vi "Target3.vi"() -> ()   [LabVIEW 2025]
uses:
  <vilib>/Platform/TimedLoop/XDataNode/timing_clust.ctl
  <vilib>/Platform/TimedLoop/XDataNode/nitl_modes.ctl
  <vilib>/Platform/TimedLoop/XDataNode/wakeup.ctl
  <vilib>/rvi/Emulation/niFpgaSctlEmulationGetInTimedLoop.vi
  <vilib>/rvi/Emulation/niFpgaEmulationReportErrorSimple.vi
  <vilib>/rvi/Emulation/niFpgaGetClockAttributes.vi
  <vilib>/rvi/Emulation/niFpgaCriticalErrorInLSC.vi
  <vilib>/rvi/linearAlgebra/MatrixMultiply/simVIs/SubVI/nifxpla_MatrixMultiply_SimMatrixSizes.vi
  <vilib>/rvi/linearAlgebra/MatrixMultiply/simVIs/SubVI/nifxpla_MatrixMultiply_Sim4WireAdapterVector.vi
  <vilib>/rvi/linearAlgebra/MatrixMultiply/simVIs/SubVI/nifxpla_MatrixMultiply_SimFrameHandShake.vi
  <vilib>/rvi/linearAlgebra/MatrixMultiply/simVIs/SubVI/nifxpla_MatrixMultiply_SimEndlessCounter.vi
  <vilib>/rvi/linearAlgebra/MatrixMultiply/simVIs/SubVI/nifxpla_MatrixMultiply_SimVectorDataBuffer.vi
  <vilib>/rvi/ClientSDK/Core/DevComputerLib/Private/Multiply(dfxp64).vi
  <vilib>/rvi/ClientSDK/Core/DevComputerLib/Private/Dfxp128ToDfxp256.vi
  <vilib>/rvi/ClientSDK/Core/DevComputerLib/Private/Add(dfxp256).vi
  <vilib>/rvi/ClientSDK/Core/DevComputerLib/Private/Subtract(dfxp256).vi
  <vilib>/rvi/ClientSDK/Core/DevComputerLib/Private/ToDfxp64(dfxp256).vi
  <vilib>/rvi/interface/RandomDataEmulation/nirviRandomDataMultiElementFPGAFIFO.vi
  <instcachedir>/0/nirviRandomDataMultiElementFPGAFIFO_BE2FF10D3D6E420AB0291A02835C249E.lvgen/nirviRandomDataMultiElementFPGAFIFO_BE2FF10D3D6E420AB0291A02835C249E_001.vi
  <vilib>/rvi/interface/RandomDataEmulation/niFpgaRandomDataHandleErrors.vi
  <vilib>/platform/TimedLoop/XDataNode/XDataNode.xnode
  <vilib>/rvi/linearAlgebra/MatrixMultiply/XNode/nifxpla_MatrixMultiply.xnode
  <vilib>/rvi/linearAlgebra/MatrixMultiply/simVIs/nifxpla_MatrixMultiply_SimTemplateEinEout.vi
  <vilib>/rvi/linearAlgebra/MatrixMultiply/simVIs/nifxpla_MatrixMultiply_SimTemplateEinVout.vi
  <vilib>/rvi/linearAlgebra/MatrixMultiply/simVIs/nifxpla_MatrixMultiply_SimTemplateVinEout.vi
  <vilib>/rvi/linearAlgebra/MatrixMultiply/simVIs/nifxpla_MatrixMultiply_SimTemplateVinVout.vi
  <vilib>/rvi/DataTransferAndStorage/Container/XNode/niFpgaContainer.xnode
  <vilib>/rvi/interface/RandomDataEmulation/nirviRandomDataFpgaMultiElementTemplate.vi
  <vilib>/Platform/TimedLoop/XDataNode/XDNodeRunTimeDep.lvlib
panel:
  out "Numeric":i32
  out "cr":fxp<+/-,32,16>[](array[numeric])
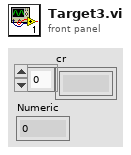
[diagram p1: front panel]
types:
  T1 = typedef "XDNodeRunTimeDep.lvlib/timing_clust.ctl" = cluster{"Expected End [f-1]":u64, "Actual End [f-1]":u64, "Finished Late? [f-1]":bool, "Expected End [i-1]":u64, "Actual End [i-1]":u64, "Finished Late? [i-1]":bool, "Expected Start [i]":u64, "Actual Start [i]":u64, "Expected Start [f]":u64, "Actual Start [f]":u64, "Source Name":string, "Structure Name":string, "Period":i64, "Deadline":i64, "Offset":i64, "Start":i64, "Priority":i32, "Timeout":i32, "Mode":T2, "Wakeup Reason":T3, "Error":errorcluster, "Source Type":string, "Secondary Source Type":string, "Global End Time":u64, "Global Start Time":u64, "Frame Duration":u64, "Iteration Duration":u64, "Assigned CPU":i32, "I/O Scan Engine Mode":u32}
  T2 = typedef "XDNodeRunTimeDep.lvlib/nitl_modes.ctl" = enum32{"No Change", "Process missed periods, maintain original phase", "Discard missed periods, maintain original phase", "Process missed periods, ignore original phase", "Discard missed periods, ignore original phase"}
  T3 = typedef "XDNodeRunTimeDep.lvlib/wakeup.ctl" = enum32{"Normal", "Aborted", "Asynchronous wakeup", "Timing source error", "Timed loop error", "Timeout"}
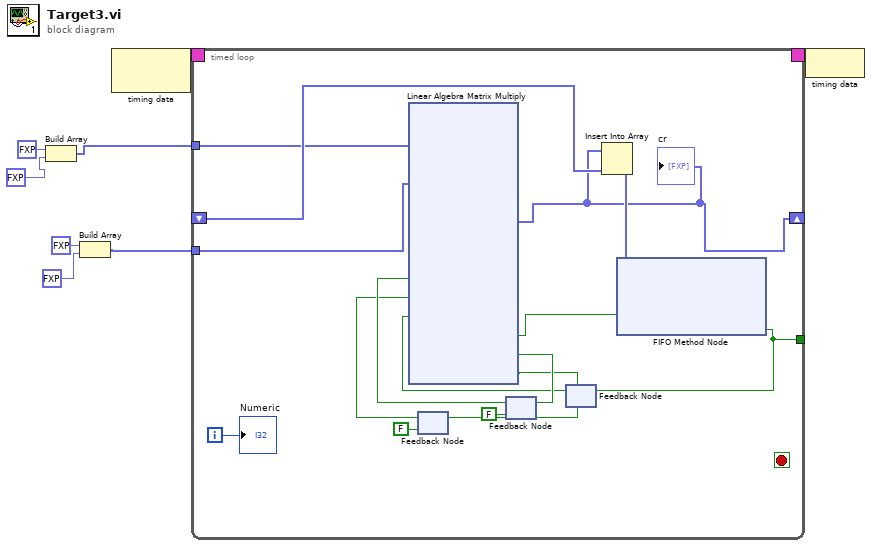
[diagram p0: block diagram]
diagram:
  n1 = Build Array(fxp<+,1,2> 2.0 ("element"), fxp<+,3,3> 5.0 ("element")) -> (w1:fxp<+,3,3>[])
  n2 = Build Array(fxp<+,2,2> 3.0 ("element"), fxp<+,2,3> 6.0 ("element")) -> (w4:fxp<+,3,3>[])
  n3 = node-c288() -> (w8:T1)  [unwired: 1 in]
  n4 = timed-loop {
    timing: w8 -> [_]
    timing-out: [_] -> w7
    tunnel: w4 -> [w17]
    shift-right: [w12] -> _
    shift-left: _ -> [w13]
    tunnel: [w11] -> _
    tunnel: w1 -> [w10]
    i -> [w9]
    stop <- _ stop-if-true
    n5 = feedback #1(FALSE ("ready for b")) -> (w20:bool)
    n6 = feedback #2(FALSE ("ready for a")) -> (w22:bool)
    n7 = feedback #3() -> (w16:bool)  [unwired: 1 in]
    n8 = xnode ("Linear Algebra Matrix Multiply")("ar"=w10, "br"=w17, "a valid"=w22, "b valid"=w20, "ready for output (T)"=w16) -> ("cr"=w12:fxp<+/-,32,16>[], "output valid"=w15:bool, "ready for a"=w23:bool, "ready for b"=w21:bool)  [unwired: 2 in, 2 out]
    "cr" <- w12
    n9 = feedback-in #1(w21) -> ()
    n10 = feedback-in #2(w23) -> ()
    n11 = Insert Into Array(array=w12, new element=w13) -> (w14:fxp<+/-,32,16>[])  [unwired: 1 in]
    n12 = xnode ("FIFO Method Node")("Element"=w14, "Input Valid"=w15) -> ("Ready for Input"=w11:bool)  [unwired: 1 in, 1 out]
    n13 = feedback-in #3(w11) -> ()
    "Numeric" <- w9
  }
  n14 = node-c288(w7) -> ()
